vi "TEST - Initialize Array to I16 Array.vi"(8 "error in (no error)":errorcluster) -> (0 "error out":errorcluster, 2 "Pass?":bool=TRUE)   [LabVIEW 2009]
doc: "This VI template can be used for the functional testing of VIs; this implementation includes handling for the testing of polymorphic VIs, and the polymorphic elements should be removed if not needed.\n\nCoded by Douglas A. Femec, January 24, 2006.\n\nCopyright (c) 2005-2006 MKS Instruments, Inc.\nAll rights reserved."
uses:
  TEST - Initialize Array from Array - Inputs.ctl
  tests/Polymorphizer+ Data Type.ctl
  TEST - Initialize Array from Array - Outputs.ctl
  Initialize Array from Array/Initialize 1D Array (I16) from 1D Array (EXT).vi
  Initialize Array from Array/Initialize 2D Array (I16) from 2D Array (EXT).vi
  Initialize Array from Array/Initialize 1D Array (I64) from 1D Array (CDB).vi
  Initialize Array from Array/Initialize 2D Array (I64) from 2D Array (CDB).vi
  Initialize Array from Array/Initialize 1D Array (I16) from 1D Array (DBL).vi
  Initialize Array from Array/Initialize 2D Array (I16) from 2D Array (DBL).vi
  Initialize Array from Array/Initialize 1D Array (I16) from 1D Array (SGL).vi
  Initialize Array from Array/Initialize 2D Array (I16) from 2D Array (SGL).vi
  Initialize Array from Array/Initialize 1D Array (I16) from 1D Array (I32).vi
  Initialize Array from Array/Initialize 2D Array (I16) from 2D Array (I32).vi
  Initialize Array from Array/Initialize 1D Array (I16) from 1D Array (I16).vi
  Initialize Array from Array/Initialize 2D Array (I16) from 2D Array (I16).vi
  Initialize Array from Array/Initialize 1D Array (I16) from 1D Array (I8).vi
  Initialize Array from Array/Initialize 2D Array (I16) from 2D Array (I8).vi
  Initialize Array from Array/Initialize 1D Array (I16) from 1D Array (U32).vi
  Initialize Array from Array/Initialize 2D Array (I16) from 2D Array (U32).vi
  Initialize Array from Array/Initialize 1D Array (I16) from 1D Array (U16).vi
  Initialize Array from Array/Initialize 2D Array (I16) from 2D Array (U16).vi
  Initialize Array from Array/Initialize 1D Array (I16) from 1D Array (U8).vi
  Initialize Array from Array/Initialize 2D Array (I16) from 2D Array (U8).vi
  Initialize Array from Array/Initialize 1D Array (I16) from 1D Array (Boolean).vi
  Initialize Array from Array/Initialize 2D Array (I16) from 2D Array (Boolean).vi
  Initialize Array from Array/Initialize 1D Array (I16) from 1D Array (String).vi
  Initialize Array from Array/Initialize 2D Array (I16) from 2D Array (String).vi
  Initialize Array from Array/Initialize 1D Array (I16) from 1D Array (Path).vi
  Initialize Array from Array/Initialize 2D Array (I16) from 2D Array (Path).vi
  Initialize Array from Array/Initialize 1D Array (I16) from 1D Array (Variant).vi
  Initialize Array from Array/Initialize 2D Array (I16) from 2D Array (Variant).vi
panel:
  out "Generated Outputs":T1[][](array[typedef]) {"1D Array" format="%.2f"; "2D Array" format="%.2f"}
  in  "Expected Outputs":T1[](array[typedef])=[{"Description"="Expect empty arrays", "1D Array"=[], "2D Array"=[]}, {"Description"="Expect 1-element arrays", "1D Array"=[1.0], "2D Array"=[[1.0]]}, {"Description"="Expect 1-row arrays", "1D Array"=[1.0], "2D Array"=[[1.0, 1.0]]}, {"Description"="Expect 1-column arrays", "1D Array"=[1.0], "2D Array"=[[1.0], [1.0], [1.0], [1.0]]}, {"Description"="Expect 2-columns, 4-rows arrays", "1D Array"=[1.0, 1.0, 1.0, 1.0], "2D Array"=[[1.0, 1.0], [1.0, 1.0], [1.0, 1.0], [1.0, 1.0]]}] {"1D Array" format="%.2f"; "2D Array" format="%.2f"}
  in  "Inputs":T2[](array[typedef])=[{"Description"="Empty arrays", "Data Types to Test"=[enum."EXT", enum."DBL", enum."SGL", enum."I32", enum."I16", enum."I8", enum."U32", enum."U16", enum."U8", enum."Boolean", enum."String", enum."Path", enum."Variant", enum."I64", enum."U64"], "1D Array"=[], "2D Array"=[]}, {"Description"="1-Element arrays", "Data Types to Test"=[enum."EXT", enum."DBL", enum."SGL", enum."I32", enum."I16", enum."I8", enum."U32", enum."U16", enum."U8", enum."Boolean", enum."String", enum."Path", enum."Variant", enum."I64", enum."U64"], "1D Array"=[1.0], "2D Array"=[[1.0]]}, {"Description"="1-Row arrays", "Data Types to Test"=[enum."EXT", enum."DBL", enum."SGL", enum."I32", enum."I16", enum."I8", enum."U32", enum."U16", enum."U8", enum."Boolean", enum."String", enum."Path", enum."Variant", enum."I64", enum."U64"], "1D Array"=[1.0], "2D Array"=[[1.0, 1.0]]}, {"Description"="1-Column arrays", "Data Types to Test"=[enum."EXT", enum."DBL", enum."SGL", enum."I32", enum."I16", enum."I8", enum."U32", enum."U16", enum."U8", enum."Boolean", enum."String", enum."Path", enum."Variant", enum."I64", enum."U64"], "1D Array"=[1.0], "2D Array"=[[1.0], [1.0], [1.0], [1.0]]}, {"Description"="2-Columns, 4-rows arrays", "Data Types to Test"=[enum."EXT", enum."DBL", enum."SGL", enum."I32", enum."I16", enum."I8", enum."U32", enum."U16", enum."U8", enum."Boolean", enum."String", enum."Path", enum."Variant", enum."I64", enum."U64"], "1D Array"=[1.0, 1.0, 1.0, 1.0], "2D Array"=[[1.0, 1.0], [1.0, 1.0], [1.0, 1.0], [1.0, 1.0]]}] {"1D Array" format="%.2f"; "2D Array" format="%.2f"}
  # "Copyright (c) 2005-2006 MKS Instruments, Inc.\nAll rights reserved."
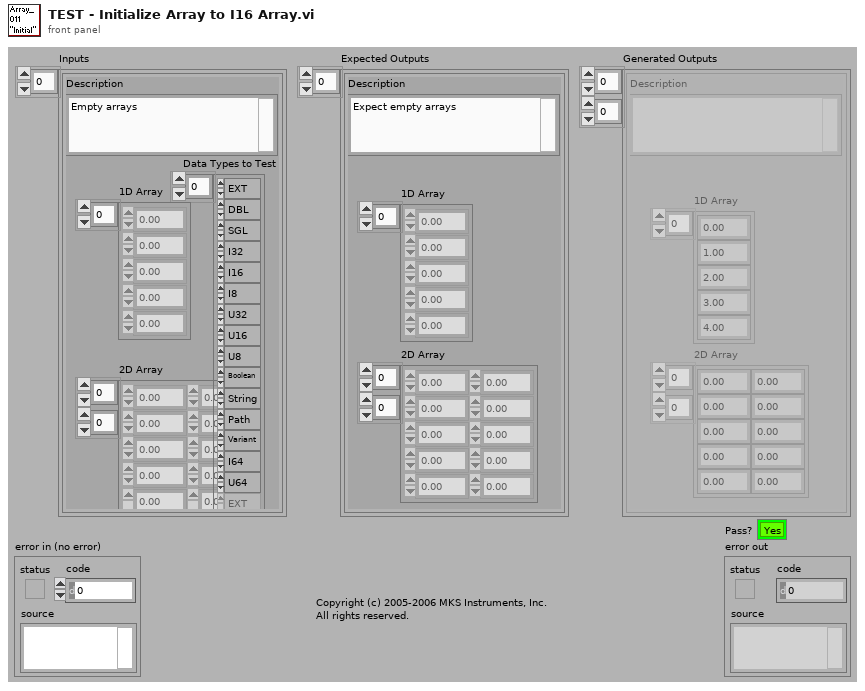
[diagram p1: front panel]
types:
  T1 = typedef "TEST - Initialize Array from Array - Outputs.ctl" = cluster{"Description":string, "1D Array":sgl[], "2D Array":sgl[][]}
  T2 = typedef "TEST - Initialize Array from Array - Inputs.ctl" = cluster{"Description":string, "Data Types to Test":T3[], "1D Array":sgl[], "2D Array":sgl[][]}
  T3 = typedef "Polymorphizer+ Data Type.ctl" = enum16{"EXT", "DBL", "SGL", "I32", "I16", "I8", "U32", "U16", "U8", "CXT", "CDB", "CSG", "Boolean", "String", "Path", "Variant", "CTL-REF", "GEN-REF", "GObj-REF", "VI-REF", "ENUM", "ERR", "FILE-REF", "MENU-REF", "MENU-RING", "PICT-RING", "TXT&PICT-RING", "TXT-RING", "I64", "U64", "LabVIEW Object"}
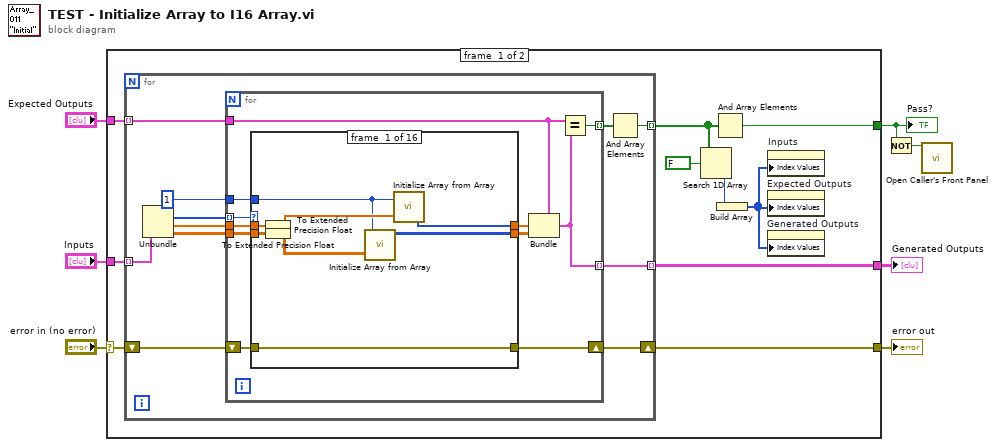
[diagram p0: block diagram]
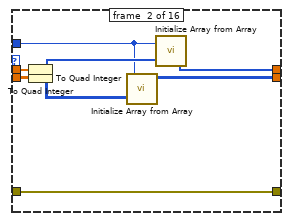
[diagram p2: hidden frame]
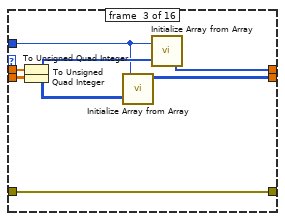
[diagram p3: hidden frame]
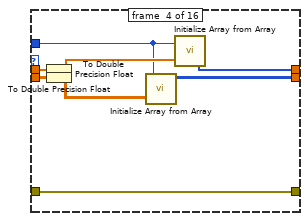
[diagram p4: hidden frame]
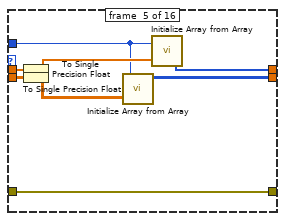
[diagram p5: hidden frame]
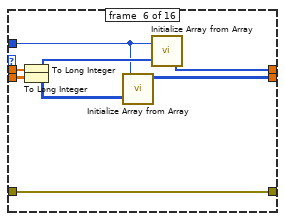
[diagram p6: hidden frame]
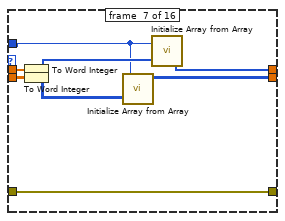
[diagram p7: hidden frame]
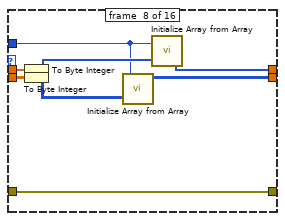
[diagram p8: hidden frame]
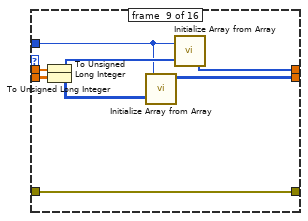
[diagram p9: hidden frame]
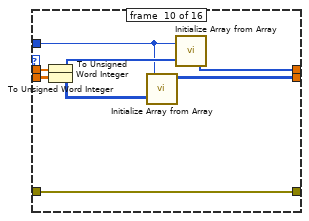
[diagram p10: hidden frame]
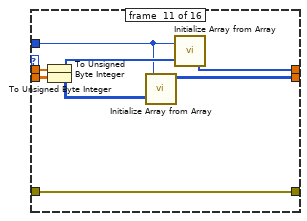
[diagram p11: hidden frame]
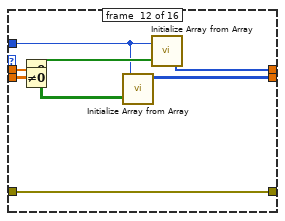
[diagram p12: hidden frame]
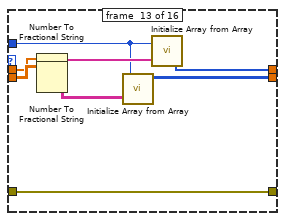
[diagram p13: hidden frame]
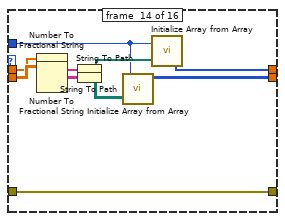
[diagram p14: hidden frame]
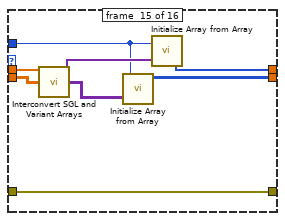
[diagram p15: hidden frame]
diagram:
  n1 = case shown="No Error" "error in (no error)" {
    selector: "error in (no error)" -> [w16 w165]
    tunnel: [w17 w165] -> w6
    tunnel: "Expected Outputs" -> [w14 _]
    tunnel: "Inputs" -> [w15 _]
    tunnel: [w13 _] -> w3
    tunnel: [w12 _] -> w1
    frame #0 {
      n2 = for {
        shift-right: [w23] -> w17
        shift-left: w16 -> [w24]
        tunnel: w15 -> [w25] mode=indexing
        tunnel: w14 -> [w28] mode=indexing
        tunnel: [w27] -> w13 mode=indexing
        tunnel: [w22] -> w11 mode=indexing
        n3 = Unbundle(w25) -> ("Data Types to Test"=w19:T3[], "1D Array"=w20:sgl[], "2D Array"=w21:sgl[][])  [unwired: 1 out]
        n4 = for {
          tunnel: w28 -> [w39]
          tunnel: [w37] -> w27 mode=indexing
          tunnel: [w38] -> w26 mode=indexing
          shift-right: [w32] -> w23
          shift-left: w24 -> [w33]
          tunnel: w19 -> [w34] mode=indexing
          tunnel: w20 -> [w36]
          tunnel: w21 -> [w35]
          tunnel: i16 1 -> [w29]
          n5 = case shown="\"U64\"" w34 {
            tunnel: w36 -> [w46 w54 w62 w70 w78 w86 w94 w102 w110 w118 w126 w134 w142 w150 w159 w163]
            tunnel: [w44 w52 w60 w68 w73 w82 w89 w97 w105 w113 w124 w129 w137 w145 w155 w163] -> w31
            tunnel: [w43 w51 w59 w65 w76 w84 w92 w100 w108 w116 w123 w128 w136 w144 w154 w162] -> w30
            tunnel: w35 -> [w47 w55 w63 w71 w79 w87 w95 w103 w111 w119 w127 w135 w143 w152 w160 w162]
            tunnel: w33 -> [w45 w53 w61 w69 w77 w85 w93 w101 w109 w117 w125 w133 w141 w149 w161 w164]
            tunnel: [w45 w53 w61 w69 w77 w85 w93 w101 w109 w117 w125 w133 w141 w149 w161 w164] -> w32
            tunnel: w29 -> [w40 w48 w56 w64 w72 w80 w88 w96 w104 w112 w120 w130 w138 w146 w156 _]
            frame #0 {
              n6 = To Extended Precision Float(1:w46) -> (0:w41:ext[])
              n7 = To Extended Precision Float(1:w47) -> (0:w42:ext[][])
              n8 = call-poly "Initialize Array from Array.vi"("Input Array"=w42, "Element Data"=w40) -> ("Output Array"=w43:i16[][])
              n9 = call-poly "Initialize Array from Array.vi"("Input Array"=w41, "Element Data"=w40) -> ("Output Array"=w44:i16[])
            }
            frame #1 {
              n10 = To Quad Integer(1:w54) -> (0:w49:i64[])
              n11 = To Quad Integer(1:w55) -> (0:w50:i64[][])
              n12 = call-poly "Initialize Array from Array.vi"("Input Array"=w50, "Element Data"=w48) -> ("Output Array"=w51:i64[][])
              n13 = call-poly "Initialize Array from Array.vi"("Input Array"=w49, "Element Data"=w48) -> ("Output Array"=w52:i64[])
            }
            frame #2 {
              n14 = To Unsigned Quad Integer(1:w62) -> (0:w57:u64[])
              n15 = To Unsigned Quad Integer(1:w63) -> (0:w58:u64[][])
              n16 = call-poly "Initialize Array from Array.vi"("Input Array"=w58, "Element Data"=w56) -> ("Output Array"=w59:i64[][])
              n17 = call-poly "Initialize Array from Array.vi"("Input Array"=w57, "Element Data"=w56) -> ("Output Array"=w60:i64[])
            }
            frame #3 {
              n18 = To Double Precision Float(number=w70) -> (double precision float=w67:dbl[])
              n19 = To Double Precision Float(number=w71) -> (double precision float=w66:dbl[][])
              n20 = call-poly "Initialize Array from Array.vi"("Input Array"=w66, "Element Data"=w64) -> ("Output Array"=w65:i16[][])
              n21 = call-poly "Initialize Array from Array.vi"("Input Array"=w67, "Element Data"=w64) -> ("Output Array"=w68:i16[])
            }
            frame #4 {
              n22 = To Single Precision Float(number=w78) -> (single precision float=w75:sgl[])
              n23 = To Single Precision Float(number=w79) -> (single precision float=w74:sgl[][])
              n24 = call-poly "Initialize Array from Array.vi"("Input Array"=w74, "Element Data"=w72) -> ("Output Array"=w76:i16[][])
              n25 = call-poly "Initialize Array from Array.vi"("Input Array"=w75, "Element Data"=w72) -> ("Output Array"=w73:i16[])
            }
            frame #5 {
              n26 = To Long Integer(number=w86) -> (32bit integer=w81:i32[])
              n27 = To Long Integer(number=w87) -> (32bit integer=w83:i32[][])
              n28 = call-poly "Initialize Array from Array.vi"("Input Array"=w83, "Element Data"=w80) -> ("Output Array"=w84:i16[][])
              n29 = call-poly "Initialize Array from Array.vi"("Input Array"=w81, "Element Data"=w80) -> ("Output Array"=w82:i16[])
            }
            frame #6 {
              n30 = To Word Integer(number=w94) -> (16bit integer=w91:i16[])
              n31 = To Word Integer(number=w95) -> (16bit integer=w90:i16[][])
              n32 = call-poly "Initialize Array from Array.vi"("Input Array"=w90, "Element Data"=w88) -> ("Output Array"=w92:i16[][])
              n33 = call-poly "Initialize Array from Array.vi"("Input Array"=w91, "Element Data"=w88) -> ("Output Array"=w89:i16[])
            }
            frame #7 {
              n34 = To Byte Integer(number=w102) -> (8bit integer=w99:i8[])
              n35 = To Byte Integer(number=w103) -> (8bit integer=w98:i8[][])
              n36 = call-poly "Initialize Array from Array.vi"("Input Array"=w98, "Element Data"=w96) -> ("Output Array"=w100:i16[][])
              n37 = call-poly "Initialize Array from Array.vi"("Input Array"=w99, "Element Data"=w96) -> ("Output Array"=w97:i16[])
            }
            frame #8 {
              n38 = To Unsigned Long Integer(number=w110) -> (unsigned 32bit integer=w107:u32[])
              n39 = To Unsigned Long Integer(number=w111) -> (unsigned 32bit integer=w106:u32[][])
              n40 = call-poly "Initialize Array from Array.vi"("Input Array"=w106, "Element Data"=w104) -> ("Output Array"=w108:i16[][])
              n41 = call-poly "Initialize Array from Array.vi"("Input Array"=w107, "Element Data"=w104) -> ("Output Array"=w105:i16[])
            }
            frame #9 {
              n42 = To Unsigned Word Integer(number=w118) -> (unsigned 16bit integer=w115:u16[])
              n43 = To Unsigned Word Integer(number=w119) -> (unsigned 16bit integer=w114:u16[][])
              n44 = call-poly "Initialize Array from Array.vi"("Input Array"=w114, "Element Data"=w112) -> ("Output Array"=w116:i16[][])
              n45 = call-poly "Initialize Array from Array.vi"("Input Array"=w115, "Element Data"=w112) -> ("Output Array"=w113:i16[])
            }
            frame #10 {
              n46 = To Unsigned Byte Integer(number=w126) -> (unsigned 8bit integer=w121:u8[])
              n47 = To Unsigned Byte Integer(number=w127) -> (unsigned 8bit integer=w122:u8[][])
              n48 = call-poly "Initialize Array from Array.vi"("Input Array"=w122, "Element Data"=w120) -> ("Output Array"=w123:i16[][])
              n49 = call-poly "Initialize Array from Array.vi"("Input Array"=w121, "Element Data"=w120) -> ("Output Array"=w124:i16[])
            }
            frame #11 {
              n50 = Not Equal To 0?(x=w134) -> (x != 0?=w132:bool[])
              n51 = Not Equal To 0?(x=w135) -> (x != 0?=w131:bool[][])
              n52 = call-poly "Initialize Array from Array.vi"("Input Array"=w131, "Element Data"=w130) -> ("Output Array"=w128:i16[][])
              n53 = call-poly "Initialize Array from Array.vi"("Input Array"=w132, "Element Data"=w130) -> ("Output Array"=w129:i16[])
            }
            frame #12 {
              n54 = Number To Fractional String(number=w142) -> (F-format string=w140:string[])  [unwired: 3 in]
              n55 = Number To Fractional String(number=w143) -> (F-format string=w139:string[][])  [unwired: 3 in]
              n56 = call-poly "Initialize Array from Array.vi"("Input Array"=w139, "Element Data"=w138) -> ("Output Array"=w136:i16[][])
              n57 = call-poly "Initialize Array from Array.vi"("Input Array"=w140, "Element Data"=w138) -> ("Output Array"=w137:i16[])
            }
            frame #13 {
              n58 = Number To Fractional String(number=w150) -> (F-format string=w151:string[])  [unwired: 3 in]
              n59 = Number To Fractional String(number=w152) -> (F-format string=w153:string[][])  [unwired: 3 in]
              n60 = String To Path(string=w151) -> (path=w148:path[])
              n61 = String To Path(string=w153) -> (path=w147:path[][])
              n62 = call-poly "Initialize Array from Array.vi"("Input Array"=w147, "Element Data"=w146) -> ("Output Array"=w144:i16[][])
              n63 = call-poly "Initialize Array from Array.vi"("Input Array"=w148, "Element Data"=w146) -> ("Output Array"=w145:i16[])
            }
            frame #14 {
              n64 = call "Interconvert SGL and Variant Arrays.vi"("SGL 1D Array In"=w159, "SGL 2D Array In"=w160) -> ("Variant 1D Array Out"=w158:variant[], "Variant 2D Array Out"=w157:variant[][])  [unwired: 9 in, 3 out]
              n65 = call-poly "Initialize Array from Array.vi"("Input Array"=w157, "Element Data"=w156) -> ("Output Array"=w154:i16[][])
              n66 = call-poly "Initialize Array from Array.vi"("Input Array"=w158, "Element Data"=w156) -> ("Output Array"=w155:i16[])
            }
            frame #15 {
            }
          }
          n67 = Bundle(cluster=w39, "1D Array"=w31, "2D Array"=w30) -> (w37:T1)  [unwired: 1 in]
          n68 = Equal?(x=w39, y=w37) -> (x = y?=w38:bool)
        }
        n69 = And Array Elements(Boolean array=w26) -> (logical AND=w22:bool)
      }
      n70 = Search 1D Array(1D array=w11, element=FALSE) -> (index of element=w9:i32)  [unwired: 1 in]
      n71 = And Array Elements(Boolean array=w11) -> (logical AND=w12:bool)
      n72 = Build Array(w9) -> (w8:i32[])
      n73 = property on="Inputs" class="Arr (strict)"("Index Values"=w8) -> ()  [unwired: 2 in, 2 out]
      n74 = property on="Expected Outputs" class="Arr (strict)"("Index Values"=w8) -> ()  [unwired: 2 in, 2 out]
      n75 = property on="Generated Outputs" class="Arr (strict)"("Index Values"=w8) -> ()  [unwired: 2 in, 2 out]
    }
    frame #1 {
    }
  }
  "error out" <- w6
  "Pass?" <- w1
  "Generated Outputs" <- w3
  n76 = Not(x=w1) -> (.not. x?=w2:bool)
  n77 = call "Open Caller's Front Panel.vi"("Open?"=w2) -> ()  [unwired: 14 in, 1 out]
